vi "Flatten to JSON Config.vi"(8 "error in (no error)":errorcluster, 11 "Tag in":refnum<class "Tag.lvclass">) -> (0 "error out":errorcluster, 2 "JSON String":string, 3 "Tag out":refnum<class "Tag.lvclass">)   [LabVIEW 2018, in "Tag Engine.lvlib" / "Tag.lvclass"]
uses:
  Tag.lvclass
  Tag.lvclass/Tag.ctl
  <vilib>/JDP Science/JSONtext/JSONtext.lvlib
  <vilib>/JDP Science/JDP Science Common Utilities/Base64/Base64 Support.lvlib
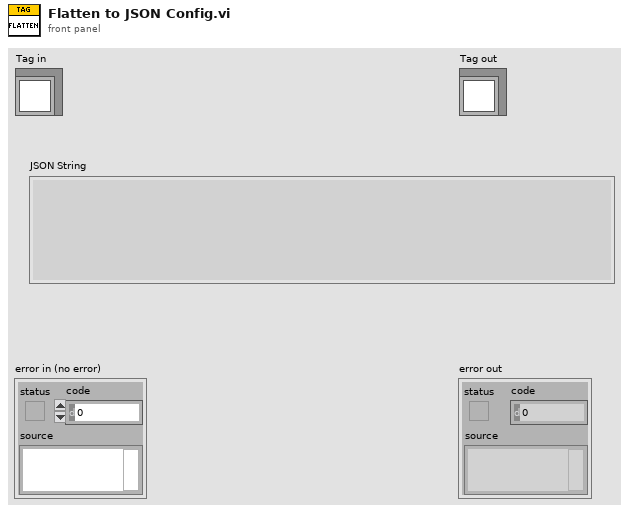
[diagram p1: front panel]
types:
  T1 = cluster{"name":string, "value":string, "typeString":i16[]}
  T2 = typedef "NI_Data Type.lvlib/Data Type.ctl" = enum8{"Invalid Type", "Void", "I8", "I16", "I32", "I64", "U8", "U16", "U32", "U64", "Single Float", "Double Float", "Extended Float", "Single Complex", "Double Complex", "Extended Complex", "Enum U8", "Enum U16", "Enum U32", "Enum U64", "Single Float With Unit", "Double Float With Unit", "Extended Float With Unit", "Single Complex with Unit", "Double Complex with Unit", "Extended Complex with Unit", "Boolean", "String", "Path", "Picture", "Tag", "Array", "Cluster", "Variant", "LV Variant", "Waveform", "Timestamp", "Digital Waveform", "Digital Data", "ExpressData", "Refnum", "External Data", "VI", "Poly VI", "LabVIEW Class Instance", "Fixed Point"}
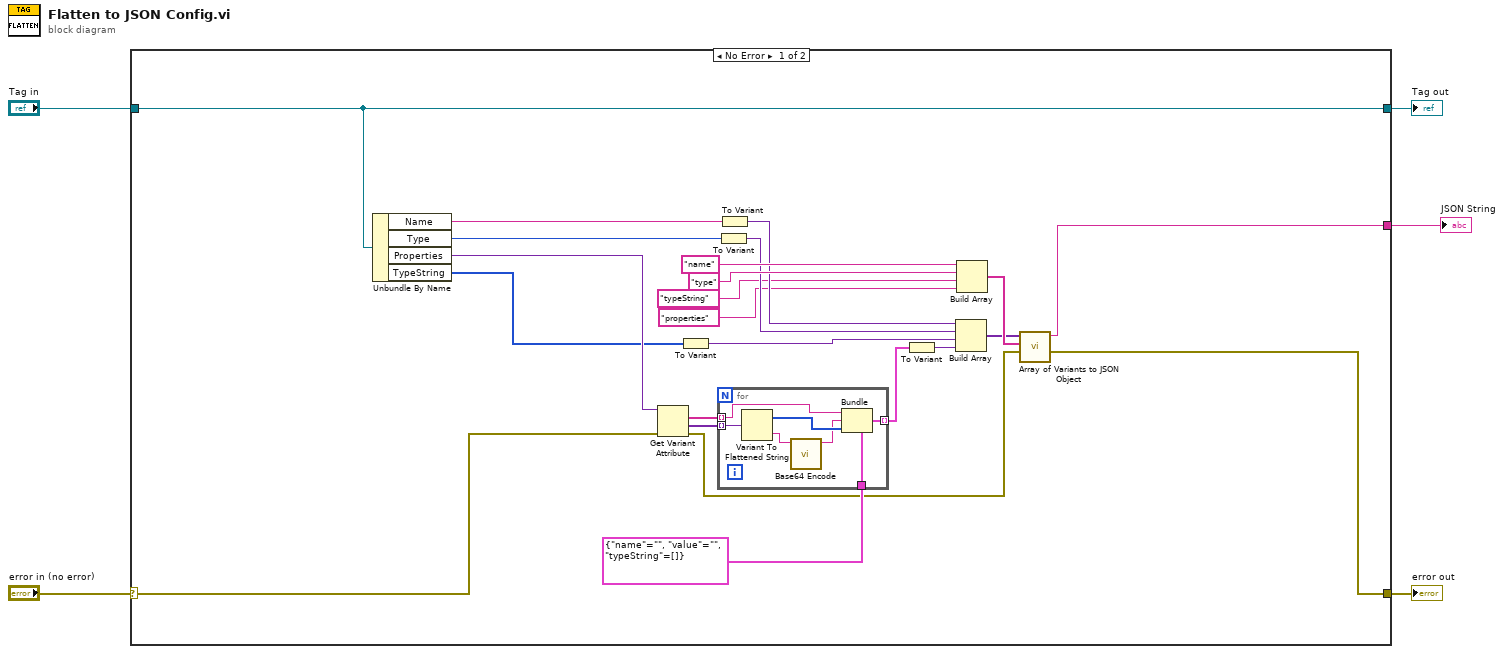
[diagram p0: block diagram]
diagram:
  n1 = case shown="No Error" "error in (no error)" {
    selector: "error in (no error)" -> [w15 w37]
    tunnel: [w17 w37] -> w4
    tunnel: [w27 w36] -> w2
    tunnel: "Tag in" -> [w27 w36]
    tunnel: [w28 _] -> w1
    frame No Error {
      n2 = Unbundle By Name(w27) -> ("Name"=w25:string, "Type"=w24:T2, "Properties"=w26:variant, "TypeString"=w16:i16[])
      n3 = Get Variant Attribute(Variant=w26, error in=w15) -> (names=w10:string[], values=w11:variant[], error out=w6:errorcluster)  [unwired: 2 in, 1 out]
      n4 = To Variant(anything=w16) -> (Variant=w13:variant)
      n5 = for {
        tunnel: w11 -> [w35] mode=indexing
        tunnel: w10 -> [w33] mode=indexing
        tunnel: T1 {"name"="", "value"="", "typeString"=[]} -> [w34]
        tunnel: [w31] -> w8 mode=indexing
        n6 = Variant To Flattened String(Variant=w35) -> (data string=w29:string, 1:w32:i16[])
        n7 = call <vilib>:"Base64 Encode.vi"("String to Encode"=w29) -> ("Base64 Encoded"=w30:string)  [unwired: 10 in]
        n8 = Bundle(cluster=w34, "name"=w33, "value"=w30, "typeString"=w32) -> (w31:T1)
      }
      n9 = To Variant(anything=w24) -> (Variant=w19:variant)
      n10 = To Variant(anything=w25) -> (Variant=w20:variant)
      n11 = To Variant(anything=w8) -> (Variant=w7:variant)
      n12 = Build Array(w20, w19, w13, w7) -> (w18:variant[])
      n13 = Build Array("name", "type", "typeString", "properties") -> (w21:string[])
      n14 = call <vilib>:"Array of Variants to JSON Object.vi"("error in (no error)"=w6, "Names"=w21, "Array"=w18) -> ("error out"=w17:errorcluster, "<JSON>"=w28:string)  [unwired: 7 in]
    }
    frame Error {
    }
  }
  "error out" <- w4
  "Tag out" <- w2
  "JSON String" <- w1
